vi "Add Comparator and Instrument Structure to Tree.vi"(6 "Add Comparator Item Tag":string, 8 "error in (no error)":errorcluster, 9 "VISA Res":refnum<visa-resource-name>, 10 "Name":string, 11 "TreeControl in":refnum<vi>) -> (0 "error out":errorcluster, 3 "reference out":refnum<vi>)   [LabVIEW 2018]
uses:
  TypeDefs/Tree Item Type.ctl
  Test Manager.lvlib
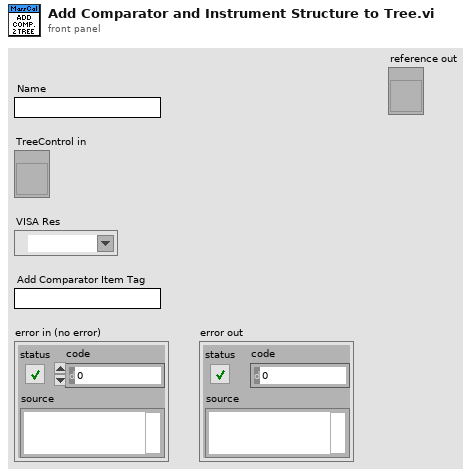
[diagram p1: front panel]
types:
  T1 = typedef "Tree Item Type.ctl" = enum16{"Comparator", "Temp Group", "Press Group", "Hygro Group", "Thermometer", "PressureTransducer", "Hygrometers", "Add Comparator", "Add Thermometer", "Add Barometer", "Add Hygrometer"}
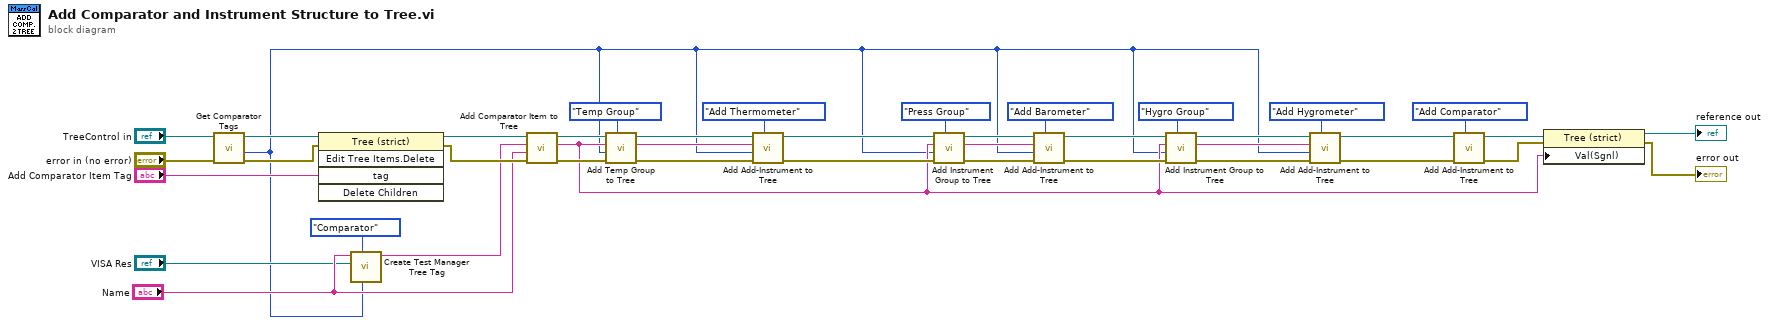
[diagram p0: block diagram]
diagram:
  n1 = call "Get Comparator Tags.vi"("error in (no error)"="error in (no error)", "TreeControl in"="TreeControl in") -> ("error out"=w24:errorcluster, "#ofComparators (New ComparatorID)"=w1:i32, "TreeControl out"=w23:refnum<vi>)  [unwired: 6 in, 1 out]
  n2 = invoke class="Tree (strict)" method="Edit Tree Items.Delete"(reference=w23, error in=w24, "tag"="Add Comparator Item Tag") -> (reference out=w36:refnum<vi>, error out=w39:errorcluster)  [unwired: 2 in, 3 out]
  n3 = call "Create Test Manager Tree Tag.vi"("Comparator ID"=w1, "ItemType"=Tree_Item_Type."Comparator", "VISA Resource"="VISA Res", "Name"="Name") -> ("Tag"=w38:string)  [unwired: 5 in, 2 out]
  n4 = call "Add Comparator Item to Tree.vi"("error in (no error)"=w39, "Name in"="Name", "Tag"=w38, "TreeControl in"=w36) -> ("error out"=w41:errorcluster, "Comparator Tag out"=w2:string, "TreeControl out"=w40:refnum<vi>)  [unwired: 5 in]
  n5 = call "Add Temp Group to Tree.vi"("ItemType"=Tree_Item_Type."Temp Group", "error in (no error)"=w41, "#ofComparators (New ComparatorID)"=w1, "Comparator Tag (Parent)"=w2, "TreeControl in"=w40) -> ("error out"=w33:errorcluster, "TempGroup Tag out"=w31:string, "TreeControl out"=w32:refnum<vi>)  [unwired: 4 in]
  n6 = call "Add Add-Instrument to Tree.vi"("ItemType"=Tree_Item_Type."Add Thermometer", "error in (no error)"=w33, "#ofComparators (New ComparatorID)"=w1, "Instrument Group Tag in"=w31, "TreeControl in"=w32) -> ("error out"=w29:errorcluster, "TreeControl out"=w28:refnum<vi>)  [unwired: 4 in, 1 out]
  n7 = call "Add Instrument Group to Tree.vi"("ItemType"=Tree_Item_Type."Press Group", "error in (no error)"=w29, "#ofComparators (New ComparatorID)"=w1, "Comparator Tag (Parent)"=w2, "TreeControl in"=w28) -> ("error out"=w30:errorcluster, "Instrument Group Tag out"=w15:string, "TreeControl out"=w16:refnum<vi>)  [unwired: 4 in]
  n8 = call "Add Add-Instrument to Tree.vi"("ItemType"=Tree_Item_Type."Add Barometer", "error in (no error)"=w30, "#ofComparators (New ComparatorID)"=w1, "Instrument Group Tag in"=w15, "TreeControl in"=w16) -> ("error out"=w17:errorcluster, "TreeControl out"=w12:refnum<vi>)  [unwired: 4 in, 1 out]
  n9 = call "Add Instrument Group to Tree.vi"("ItemType"=Tree_Item_Type."Hygro Group", "error in (no error)"=w17, "#ofComparators (New ComparatorID)"=w1, "Comparator Tag (Parent)"=w2, "TreeControl in"=w12) -> ("error out"=w13:errorcluster, "Instrument Group Tag out"=w7:string, "TreeControl out"=w10:refnum<vi>)  [unwired: 4 in]
  n10 = call "Add Add-Instrument to Tree.vi"("ItemType"=Tree_Item_Type."Add Hygrometer", "error in (no error)"=w13, "#ofComparators (New ComparatorID)"=w1, "Instrument Group Tag in"=w7, "TreeControl in"=w10) -> ("error out"=w11:errorcluster, "TreeControl out"=w5:refnum<vi>)  [unwired: 4 in, 1 out]
  n11 = call "Add Add-Instrument to Tree.vi"("ItemType"=Tree_Item_Type."Add Comparator", "error in (no error)"=w11, "TreeControl in"=w5) -> ("error out"=w6:errorcluster, "TreeControl out"=w4:refnum<vi>)  [unwired: 6 in, 1 out]
  n12 = property class="Tree (strict)"(reference=w4, error in=w6, "Val(Sgnl)"=w2) -> (reference out=→"reference out":refnum<vi>, error out=→"error out":errorcluster)
